vi "3D-CollectSegmentName.vi"(11 "Chose Porgram":string(combo)) -> (0 "SegmentPos":string[][](array[string]), 1 "StepNubner":i32, 3 "SegmentName":string[](array[string]))   [LabVIEW 2015]
uses:
  Global System.vi
  <vilib>/Utility/file.llb/Read From Spreadsheet File (string).vi
panel:
  out "StepNubner":string
  out "已删除元素的数组子集":string[][](array[string])
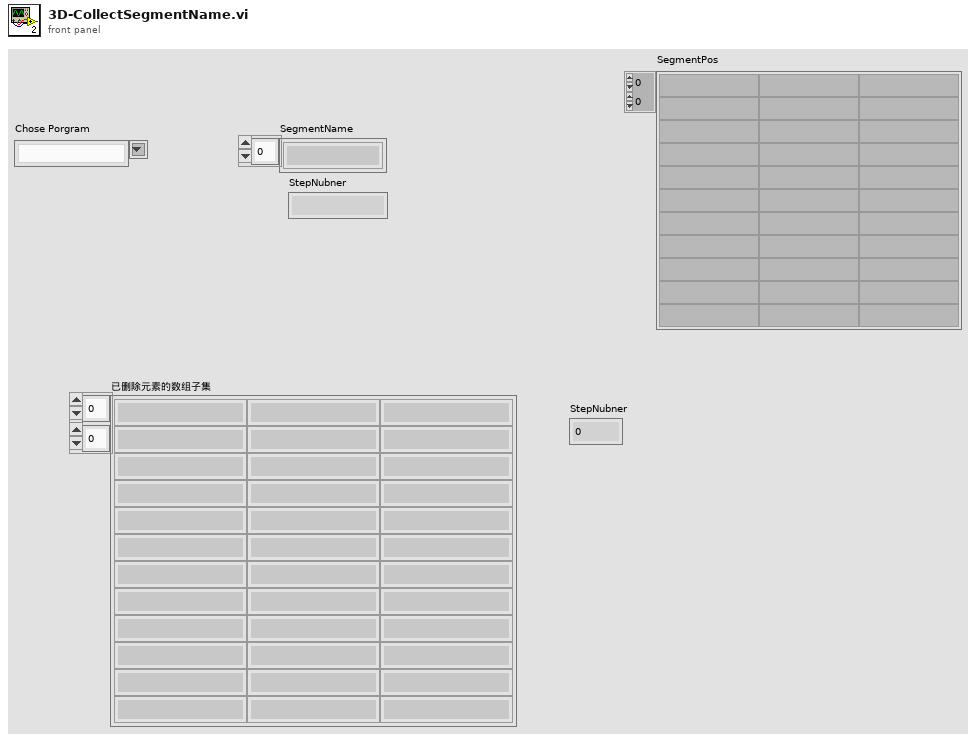
[diagram p1: front panel]
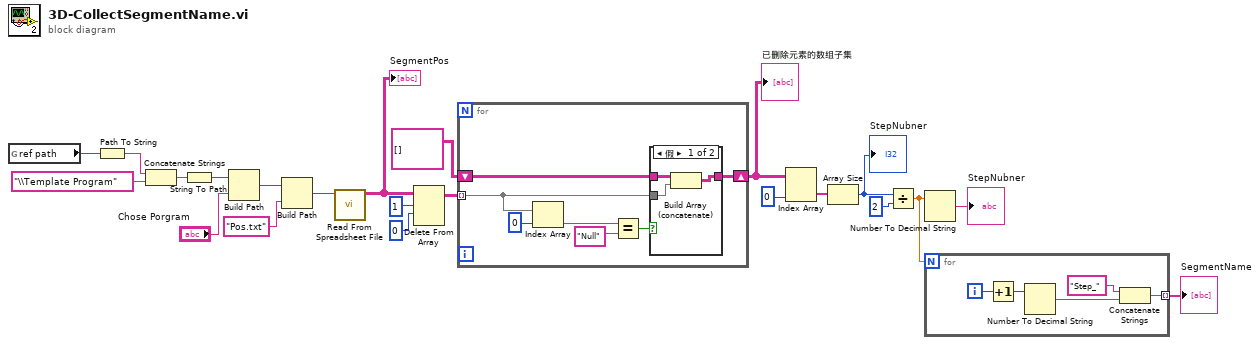
[diagram p0: block diagram]
diagram:
  n1 = global read "Global System.vi" "ref path"() -> (w22:path)
  n2 = Path To String(path=w22) -> (string=w19:string)
  n3 = Concatenate Strings(w19, "\\Template Program" ("字符串")) -> (w21:string)
  n4 = String To Path(string=w21) -> (path=w16:path)
  n5 = Build Path(base path=w16, name or relative path="Chose Porgram") -> (appended path=w17:path)
  n6 = Build Path(base path=w17, name or relative path="Pos.txt" ("名称或相对路径")) -> (appended path=w14:path)
  n7 = call-poly <vilib>:"Read From Spreadsheet File.vi"("file path (dialog if empty)"=w14) -> ("all rows"=w13:string[][])  [unwired: 6 in, 4 out]
  "SegmentPos" <- w13
  n8 = Delete From Array(array=w13, length=1 ("长度"), index (row)=0 ("索引 (行)")) -> (array with subset deleted=w3:string[][])  [unwired: 1 in, 1 out]
  n9 = for {
    shift-right: [w24] -> w1
    shift-left: string[][] [] -> [w25]
    tunnel: w3 -> [w23] mode=indexing
    n10 = Index Array(array=w23, index=0 ("索引")) -> (element=w28:string)
    n11 = Equal?(x=w28, y="Null") -> (x = y?=w26:bool)
    n12 = case shown="假" w26 {
      tunnel: w25 -> [w32 w33]
      tunnel: [w31 w33] -> w24
      tunnel: w23 -> [w30 _]
      frame False {
        n13 = Build Array (concatenate)(w32, w30) -> (w31:string[][])
      }
      frame True {
      }
    }
  }
  "已删除元素的数组子集" <- w1
  n14 = Index Array(array=w1, index (col)=0 ("禁用的索引 (列)")) -> (element=w9:string[])  [unwired: 1 in]
  n15 = Array Size(array=w9) -> (size(s)=w8:i32)
  "StepNubner" <- w8
  n16 = Divide(x=w8, y=2) -> (x/y=w5:dbl)
  n17 = Number To Decimal String(number=w5) -> (decimal integer string=→"StepNubner":string)  [unwired: 1 in]
  n18 = for {
    N: w5 -> [_]
    tunnel: [w34] -> w6 mode=indexing
    i -> [w37]
    n19 = Increment(x=w37) -> (x+1=w36:i32)
    n20 = Number To Decimal String(number=w36) -> (decimal integer string=w35:string)  [unwired: 1 in]
    n21 = Concatenate Strings("Step_", w35) -> (w34:string)
  }
  "SegmentName" <- w6
